vi "Begin.vi"(8 "error in":errorcluster) -> (0 "error out":errorcluster)   [LabVIEW 2019]
doc: "Called before other user functions, this VI can be used to open I/O refnums, load in file data, and do general program initialization. Notice that the <B>error out</B> terminal is simply used for data flow. Wiring it to other structures or subVIs ensures that this VI runs first."
uses:
  <vilib>/Rock Robotics/WPI/DriverStation/WPI_DriverStationRobotMode2.ctl
  <vilib>/Rock Robotics/WPI/Joystick/WPI_JoystickDeviceEnum.ctl
  <vilib>/Rock Robotics/SystemInterfaces/DIO/FPGA_DIOPWMChannel.ctl
  <vilib>/Rock Robotics/WPI/SafetyOutput/WPI_SafetyOutputConfigMenu.ctl
  <vilib>/Rock Robotics/WPI/Solenoid/WPI_SolenoidChannel.ctl
  <vilib>/Rock Robotics/SystemInterfaces/i2clib/i2c_bus.ctl
  <vilib>/Rock Robotics/WPI/Solenoid/WPI_SolenoidValue.ctl
  Robot Global Data.vi
  <vilib>/Rock Robotics/WPI/RobotDrive/WPI_RobotDriveOpen2MotorWithExistingMotors.vi
  <vilib>/Rock Robotics/WPI/MotorControl/WPI_MotorControlOpen SPARK.vi
  <vilib>/Rock Robotics/WPI/Solenoid/WPI_SolenoidOpenDouble.vi
  <vilib>/Rock Robotics/WPI/Solenoid/WPI_SolenoidSetEnum.vi
  <vilib>/Rock Robotics/Network Tables/NT Write Number.vi
  <vilib>/Rock Robotics/Network Tables/NT Write Boolean Array.vi
  <vilib>/Rock Robotics/Network Tables/NT Write Numeric Array.vi
panel:
  in  "Calibration Time (sec)":u32=4
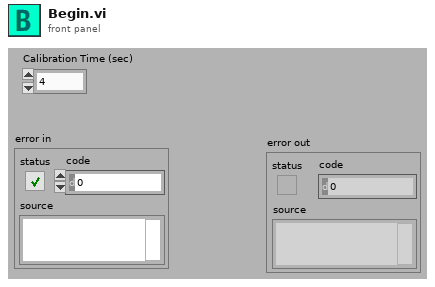
[diagram p1: front panel]
types:
  T1 = typedef "WPI_SolenoidChannel.ctl" = enum8{"Solenoid 0", "Solenoid 1", "Solenoid 2", "Solenoid 3", "Solenoid 4", "Solenoid 5", "Solenoid 6", "Solenoid 7", "Invalid"}
  T2 = typedef "WPI_SolenoidValue.ctl" = enum16{"Off", "On", "Forward", "Reverse"}
  T3 = typedef "WPI_SafetyOutputConfigMenu.ctl" = enum16{"Enable", "Disable"}
  T4 = typedef "i2c_bus.ctl" = enum16{"I2C On-Board", "I2C MXP", "Invalid"}
  T5 = typedef "FPGA_DIOPWMChannel.ctl" = enum8{"PWM 0", "PWM 1", "PWM 2", "PWM 3", "PWM 4", "PWM 5", "PWM 6", "PWM 7", "PWM 8", "PWM 9", "PWM MXP 0", "PWM MXP 1", "PWM MXP 2", "PWM MXP 3", "PWM MXP 4", "PWM MXP 5", "PWM MXP 6", "PWM MXP 7", "PWM MXP 8", "PWM MXP 9", "Invalid"}
  T6 = typedef "WPI_JoystickDeviceEnum.ctl" = enum16{"USB 0", "USB 1", "USB 2", "USB 3", "USB 4", "USB 5"}
  T7 = typedef "WPI_DriverStationRobotMode2.ctl" = enum16{"Autonomous Disabled", "Autonomous Enabled", "Teleop Disabled", "Teleop Enabled", "Disconnected", "Finish", "Test Disabled", "Test Enabled", "Emergency Stopped"}
  T8 = typedef "WPI_JoystickDevRef.ctl" = cluster{"Device":T6}
  T9 = typedef "WPI_MotorControlDeviceRef.ctl" = cluster{"DeviceStatus":errorcluster, "Type":T10, "PWM":cluster{"PWM Channel":T5, "DeadBand":T11}, "CAN":cluster{"Device Number":u8, "SetOutput VI Ref":variant, "GetOutput VI Ref":variant, "Enable VI Ref":variant, "Disable VI Ref":variant, "Data":variant}, "Invert":bool, "DIO PWM":cluster{"PWM \"Enable\" Channel":T5, "DIOChannel":T12, "PWM Rate":dbl}}
  T10 = typedef "WPI_MotorControlType.ctl" = enum16{"PWM", "CAN", "DIO PWM"}
  T11 = typedef "WPI_PWMDeadband.ctl" = cluster{"Name":string, "maxPositivePwm":i32, "minPositivePwm":i32, "centerPwm":i32, "maxNegativePwm":i32, "minNegativePwm":i32, "angularRange":u16}
  T12 = typedef "FPGA_DIOChannel.ctl" = enum8{"DIO 0", "DIO 1", "DIO 2", "DIO 3", "DIO 4", "DIO 5", "DIO 6", "DIO 7", "DIO 8", "DIO 9", "DIO MXP 0", "DIO MXP 1", "DIO MXP 2", "DIO MXP 3", "DIO MXP 4", "DIO MXP 5", "DIO MXP 6", "DIO MXP 7", "DIO MXP 8", "DIO MXP 9", "DIO MXP 10", "DIO MXP 11", "DIO MXP 12", "DIO MXP 13", "DIO MXP 14", "DIO MXP 15", "SPI Port CS1", "SPI Port CS2", "SPI Port CS3", "SPI Port MISO", "SPI Port MOSI", "Invalid"}
  T13 = typedef "WPI_RobotDriveDevRef.ctl" = cluster{"DevStatus":errorcluster, "Motors[]":T9[], "Square Inputs":bool, "Max Output":dbl}
  T14 = typedef "ADIS 16448 HW Configuration.ctl" = cluster{"SPI Clock Rate (Hz)":dbl, "IMU SPI Mode (3)":T15, "IMU Reset Pin":T12, "IMU SPI Bus":T16, "IMU Data Ready Pin":T12, "Stall Config":cluster{"Pow2BytesPerRead":u8, "StallTicks":u16, "CsToSclkTicks":u8}, "IMU Status LED Pin":T12}
  T15 = typedef "WPI_SPIMode.ctl" = enum16{"Mode 0 (Clk Idle Low,Sample on Leading)", "Mode 1 (Clk Idle Low,Sample on Trailing)", "Mode 2 (Clk Idle High,Sample on Leading)", "Mode 3 (Clk Idle High,Sample on Trailing)"}
  T16 = typedef "spi_bus.ctl" = enum16{"SPI On-Board, CS0", "SPI On-Board, CS1", "SPI On-Board, CS2", "SPI On-Board, CS3", "SPI MXP", "Invalid"}
  T17 = typedef "ADIS16448 Device Reference.ctl" = cluster{"DevStatus":errorcluster, "Hardware Config":T18, "Calibration Complete":refnum<notifier>, "Status FIFO":refnum<k33>, "Last Value Reference":refnum<data-value>, "Sychronous Process VI":T19, "Cmd FIFO":refnum<k33>, "Source":T20, "Data FIFO":refnum<k33>, "IMU Status LED Pin":T12, "Calibration Time":u32}
  T18 = typedef "ADIS16448 Hardware Configuration.ctl" = cluster{"SPI Clock Rate (Hz)":dbl, "IMU SPI Mode (3)":T15, "IMU Reset Pin":T12, "IMU SPI Bus":T16, "IMU Data Ready Pin":T12, "Stall Config":cluster{"Pow2BytesPerRead":u8, "StallTicks":u16, "CsToSclkTicks":u8}, "IMU Status LED Pin":T12}
  T19 = typedef "ADIS16448 Process.ctl" = refnum<vi>
  T20 = typedef "FPGA_CounterEncoderSourceConvertionLVSourceType.ctl" = cluster{"DevStatus":errorcluster, "AnalogTriggerMode?":bool, "DigitalMode":cluster{"DIO Channel":T21}, "AnalogTriggerMode":cluster{"AnalogTriggerIndex":T22, "OutputType":T23}}
  T21 = typedef "FPGA_DIODigitalSourceChannel.ctl" = enum8{"DIO 0", "DIO 1", "DIO 2", "DIO 3", "DIO 4", "DIO 5", "DIO 6", "DIO 7", "DIO 8", "DIO 9", "DIO MXP 0", "DIO MXP 1", "DIO MXP 2", "DIO MXP 3", "DIO MXP 4", "DIO MXP 5", "DIO MXP 6", "DIO MXP 7", "DIO MXP 8", "DIO MXP 9", "DIO MXP 10", "DIO MXP 11", "DIO MXP 12", "DIO MXP 13", "DIO MXP 14", "DIO MXP 15", "SPI Port CS1", "SPI Port CS2", "SPI Port CS3", "SPI Port MISO", "SPI Port MOSI", "Disabled"}
  T22 = typedef "FPGA_AnalogTriggerIndex.ctl" = enum8{"Trig 0", "Trig 1", "Trig 2", "Trig 3", "Trig 4", "Trig 5", "Trig 6", "Trig 7", "Invalid"}
  T23 = typedef "FPGA_AnalogTriggerOutType.ctl" = enum16{"InWindow", "TriggerState", "Rising", "Falling"}
  T24 = typedef "Color Sensor V3 DevRef.ctl" = cluster{"I2CDevRef":T25}
  T25 = typedef "WPI_I2CDevRef.ctl" = cluster{"DevStatus":errorcluster, "Device Address":u8, "Handle":i32, "I2C Bus":T4}
  T26 = typedef "WPI_SolenoidDevRef.ctl" = cluster{"DevStatus":errorcluster, "Pneumatics Control Module":u8, "Forward Solenoid Channel":T1, "Reverse Solenoid Channel":T1}
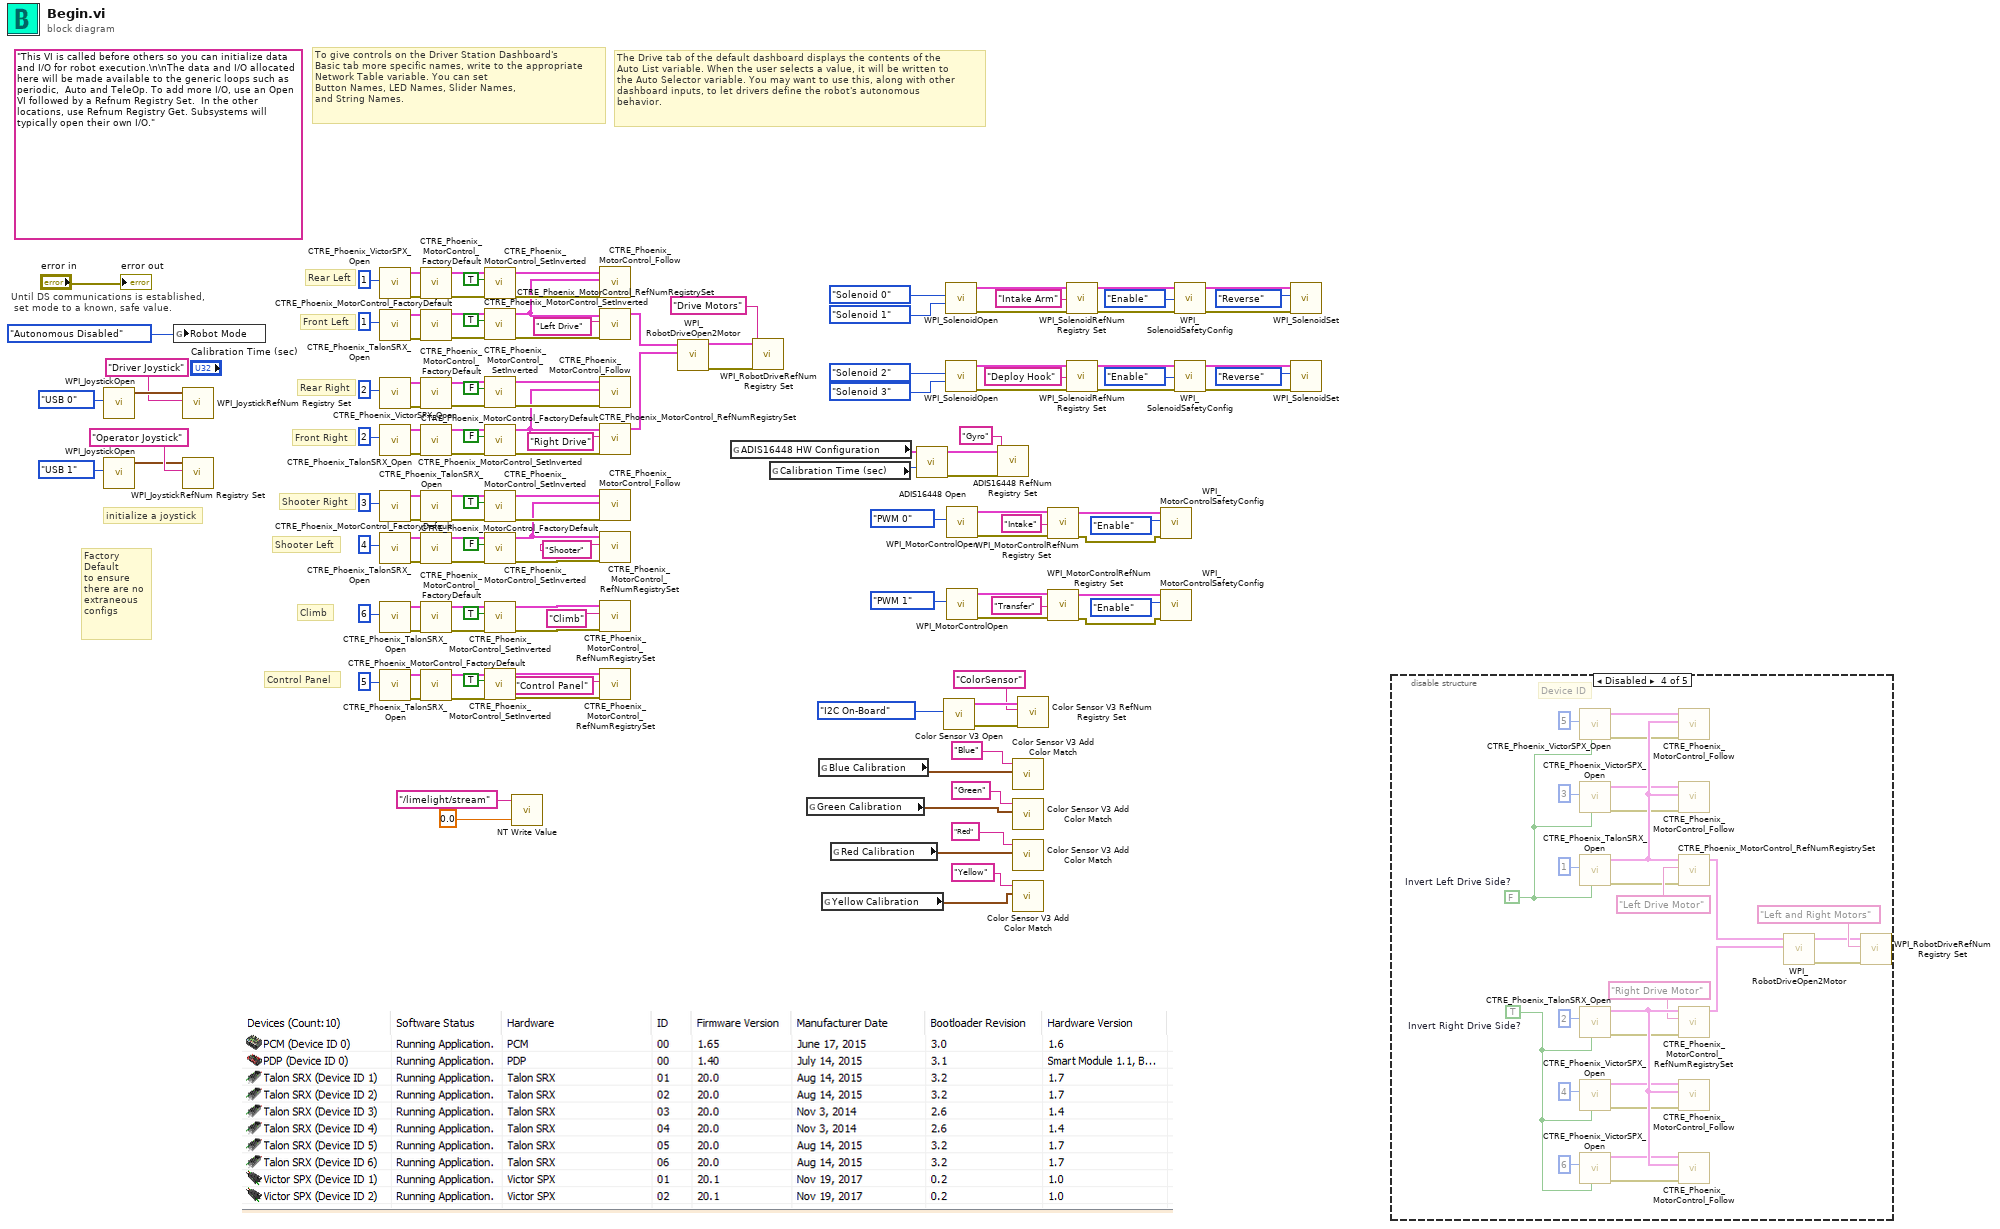
[diagram p0: block diagram]
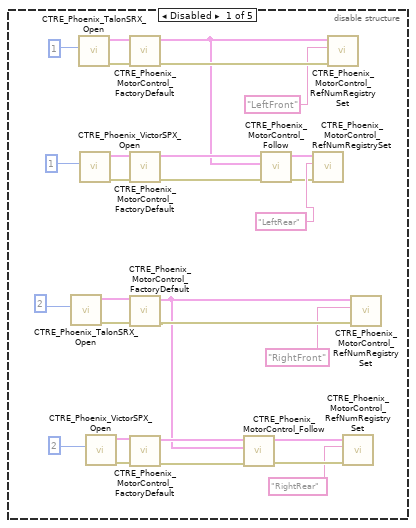
[diagram p2: hidden frame]
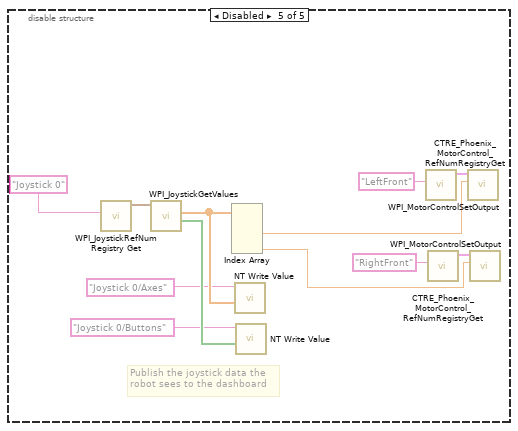
[diagram p5: hidden frame]
diagram:
  (unwired) "This VI is called before others so you can initialize data and I/O for robot execution.\n\nThe data and I/O allocated here will be made available to the generic loops such as periodic,  Auto and TeleOp. To add more I/O, use an Open VI followed by a Refnum Registry Set.  In the other locations, use Refnum Registry Get. Subsystems will typically open their own I/O."
  # "Climb"
  # "Control Panel"
  # "The Drive tab of the default dashboard displays the contents of the\nAuto List variable. When the user selects a value, it will be written to\nthe Auto Selector variable. You may want to use this, along with other\ndashboard inputs, to let drivers define the robot's autonomous\nbehavior."
  # "To give controls on the Driver Station Dashboard's\nBasic tab more specific names, write to the appropriate\nNetwork Table variable. You can set\nButton Names, LED Names, Slider Names,\nand String Names."
  # "Shooter Left"
  # "Shooter Right"
  # "Factory \nDefault \nto ensure \nthere are no \nextraneous \nconfigs"
  # "Front Right"
  # "Front Left"
  # "Rear Right"
  # "Rear Left"
  # "initialize a joystick"
  # "Until DS communications is established,\n set mode to a known, safe value."
  n1 = call <vilib>:"WPI_JoystickOpen.vi"("JoystickDevice"=WPI_JoystickDeviceEnum."USB 0") -> ("JoystickDevRef"=w120:T8)  [unwired: 10 in]
  n2 = call <vilib>:"WPI_JoystickOpen.vi"("JoystickDevice"=WPI_JoystickDeviceEnum."USB 1") -> ("JoystickDevRef"=w135:T8)  [unwired: 10 in]
  n3 = global write "Robot Global Data.vi" "Robot Mode"(WPI_DriverStationRobotMode2."Autonomous Disabled" ("Robot Mode")) -> ()
  n4 = call <vilib>:"WPI_JoystickRefNum Registry Set.vi"("refnum name"="Driver Joystick", "JoystickDevRef"=w120) -> ()  [unwired: 8 in, 2 out]
  n5 = call <vilib>:"WPI_JoystickRefNum Registry Set.vi"("refnum name"="Operator Joystick", "JoystickDevRef"=w135) -> ()  [unwired: 8 in, 2 out]
  n6 = call <vilib>:"CTRE_Phoenix_VictorSPX_Open.vi"("Device Number"=u8 1) -> ("error out"=w118:errorcluster, "CAN Talon SRX Ref"=w117:T9)  [unwired: 9 in]
  n7 = call <vilib>:"CTRE_Phoenix_TalonSRX_Open.vi"("Device Number"=u8 1) -> ("error out"=w115:errorcluster, "CAN Talon SRX Ref"=w116:T9)  [unwired: 9 in]
  n8 = call <vilib>:"CTRE_Phoenix_VictorSPX_Open.vi"("Device Number"=u8 2) -> ("error out"=w114:errorcluster, "CAN Talon SRX Ref"=w113:T9)  [unwired: 9 in]
  n9 = call <vilib>:"CTRE_Phoenix_TalonSRX_Open.vi"("Device Number"=u8 2) -> ("error out"=w112:errorcluster, "CAN Talon SRX Ref"=w111:T9)  [unwired: 9 in]
  n10 = call <vilib>:"CTRE_Phoenix_TalonSRX_Open.vi"("Device Number"=u8 3) -> ("error out"=w73:errorcluster, "CAN Talon SRX Ref"=w72:T9)  [unwired: 9 in]
  n11 = call <vilib>:"CTRE_Phoenix_TalonSRX_Open.vi"("Device Number"=u8 4) -> ("error out"=w71:errorcluster, "CAN Talon SRX Ref"=w70:T9)  [unwired: 9 in]
  n12 = call <vilib>:"CTRE_Phoenix_TalonSRX_Open.vi"("Device Number"=u8 6) -> ("error out"=w11:errorcluster, "CAN Talon SRX Ref"=w10:T9)  [unwired: 9 in]
  n13 = call <vilib>:"CTRE_Phoenix_TalonSRX_Open.vi"("Device Number"=u8 5) -> ("error out"=w41:errorcluster, "CAN Talon SRX Ref"=w40:T9)  [unwired: 9 in]
  n14 = call <vilib>:"CTRE_Phoenix_MotorControl_FactoryDefault.vi"("error in"=w118, "PhoenixMotorControlDevRef"=w117) -> ("error out"=w109:errorcluster, "PhoenixMotorControlDevRef"=w108:T9)  [unwired: 8 in]
  n15 = call <vilib>:"CTRE_Phoenix_MotorControl_FactoryDefault.vi"("error in"=w115, "PhoenixMotorControlDevRef"=w116) -> ("error out"=w103:errorcluster, "PhoenixMotorControlDevRef"=w104:T9)  [unwired: 8 in]
  n16 = call <vilib>:"CTRE_Phoenix_MotorControl_FactoryDefault.vi"("error in"=w114, "PhoenixMotorControlDevRef"=w113) -> ("error out"=w99:errorcluster, "PhoenixMotorControlDevRef"=w98:T9)  [unwired: 8 in]
  n17 = call <vilib>:"CTRE_Phoenix_MotorControl_FactoryDefault.vi"("error in"=w112, "PhoenixMotorControlDevRef"=w111) -> ("error out"=w94:errorcluster, "PhoenixMotorControlDevRef"=w93:T9)  [unwired: 8 in]
  n18 = call <vilib>:"CTRE_Phoenix_MotorControl_FactoryDefault.vi"("error in"=w73, "PhoenixMotorControlDevRef"=w72) -> ("error out"=w67:errorcluster, "PhoenixMotorControlDevRef"=w68:T9)  [unwired: 8 in]
  n19 = call <vilib>:"CTRE_Phoenix_MotorControl_FactoryDefault.vi"("error in"=w71, "PhoenixMotorControlDevRef"=w70) -> ("error out"=w62:errorcluster, "PhoenixMotorControlDevRef"=w63:T9)  [unwired: 8 in]
  n20 = call <vilib>:"CTRE_Phoenix_MotorControl_FactoryDefault.vi"("error in"=w11, "PhoenixMotorControlDevRef"=w10) -> ("error out"=w7:errorcluster, "PhoenixMotorControlDevRef"=w8:T9)  [unwired: 8 in]
  n21 = call <vilib>:"CTRE_Phoenix_MotorControl_FactoryDefault.vi"("error in"=w41, "PhoenixMotorControlDevRef"=w40) -> ("error out"=w37:errorcluster, "PhoenixMotorControlDevRef"=w38:T9)  [unwired: 8 in]
  n22 = call <vilib>:"CTRE_Phoenix_MotorControl_SetInverted.vi"("error in (no error)"=w109, "Invert?"=TRUE, "PhoenixMotorControlDevRef"=w108) -> ("error out"=w106:errorcluster, "PhoenixMotorControlDevRef"=w107:T9)  [unwired: 7 in]
  n23 = call <vilib>:"CTRE_Phoenix_MotorControl_SetInverted.vi"("error in (no error)"=w103, "Invert?"=TRUE, "PhoenixMotorControlDevRef"=w104) -> ("error out"=w102:errorcluster, "PhoenixMotorControlDevRef"=w101:T9)  [unwired: 7 in]
  n24 = call <vilib>:"CTRE_Phoenix_MotorControl_SetInverted.vi"("error in (no error)"=w99, "Invert?"=FALSE, "PhoenixMotorControlDevRef"=w98) -> ("error out"=w96:errorcluster, "PhoenixMotorControlDevRef"=w97:T9)  [unwired: 7 in]
  n25 = call <vilib>:"CTRE_Phoenix_MotorControl_SetInverted.vi"("error in (no error)"=w94, "Invert?"=FALSE, "PhoenixMotorControlDevRef"=w93) -> ("error out"=w91:errorcluster, "PhoenixMotorControlDevRef"=w92:T9)  [unwired: 7 in]
  n26 = call <vilib>:"CTRE_Phoenix_MotorControl_SetInverted.vi"("error in (no error)"=w67, "Invert?"=TRUE, "PhoenixMotorControlDevRef"=w68) -> ("error out"=w66:errorcluster, "PhoenixMotorControlDevRef"=w65:T9)  [unwired: 7 in]
  n27 = call <vilib>:"CTRE_Phoenix_MotorControl_SetInverted.vi"("error in (no error)"=w62, "Invert?"=FALSE, "PhoenixMotorControlDevRef"=w63) -> ("error out"=w61:errorcluster, "PhoenixMotorControlDevRef"=w60:T9)  [unwired: 7 in]
  n28 = call <vilib>:"CTRE_Phoenix_MotorControl_SetInverted.vi"("error in (no error)"=w7, "Invert?"=TRUE, "PhoenixMotorControlDevRef"=w8) -> ("error out"=w6:errorcluster, "PhoenixMotorControlDevRef"=w5:T9)  [unwired: 7 in]
  n29 = call <vilib>:"CTRE_Phoenix_MotorControl_SetInverted.vi"("error in (no error)"=w37, "Invert?"=TRUE, "PhoenixMotorControlDevRef"=w38) -> ("error out"=w36:errorcluster, "PhoenixMotorControlDevRef"=w35:T9)  [unwired: 7 in]
  n30 = call-poly <vilib>:"NT Write Value.vi"("Numeric"=0.0, "Name"="/limelight/stream") -> ()  [unwired: 9 in, 1 out]
  n31 = call <vilib>:"CTRE_Phoenix_MotorControl_Follow.vi"("error in (no error)"=w106, "Master Controller to Follow"=w101, "PhoenixMotorControlDevRef"=w107) -> ()  [unwired: 7 in, 2 out]
  n32 = call <vilib>:"CTRE_Phoenix_MotorControl_RefNumRegistrySet.vi"("error in (no error)"=w102, "refnum name"="Left Drive", "PhoenixMotorControlDevRef"=w101) -> ("PhoenixMotorControlDevRef"=w128:T9)  [unwired: 7 in, 1 out]
  n33 = call <vilib>:"CTRE_Phoenix_MotorControl_Follow.vi"("error in (no error)"=w96, "Master Controller to Follow"=w92, "PhoenixMotorControlDevRef"=w97) -> ()  [unwired: 7 in, 2 out]
  n34 = call <vilib>:"CTRE_Phoenix_MotorControl_RefNumRegistrySet.vi"("error in (no error)"=w91, "refnum name"="Right Drive", "PhoenixMotorControlDevRef"=w92) -> ("PhoenixMotorControlDevRef"=w127:T9)  [unwired: 7 in, 1 out]
  n35 = call <vilib>:"CTRE_Phoenix_MotorControl_Follow.vi"("error in (no error)"=w66, "Master Controller to Follow"=w60, "PhoenixMotorControlDevRef"=w65) -> ()  [unwired: 7 in, 2 out]
  n36 = call <vilib>:"CTRE_Phoenix_MotorControl_RefNumRegistrySet.vi"("error in (no error)"=w61, "refnum name"="Shooter", "PhoenixMotorControlDevRef"=w60) -> ()  [unwired: 7 in, 2 out]
  n37 = call <vilib>:"CTRE_Phoenix_MotorControl_RefNumRegistrySet.vi"("error in (no error)"=w6, "refnum name"="Climb", "PhoenixMotorControlDevRef"=w5) -> ()  [unwired: 7 in, 2 out]
  n38 = call <vilib>:"CTRE_Phoenix_MotorControl_RefNumRegistrySet.vi"("error in (no error)"=w36, "refnum name"="Control Panel", "PhoenixMotorControlDevRef"=w35) -> ()  [unwired: 7 in, 2 out]
  n39 = call-poly <vilib>:"WPI_RobotDriveOpen2Motor.vi"("Right Motor Dev Ref"=w127, "Left Motor Dev Ref"=w128) -> ("error out"=w123:errorcluster, "RobotDriveDevRef"=w124:T13)  [unwired: 8 in]
  n40 = global read "Robot Global Data.vi" "ADIS16448 HW Configuration"() -> (w59:T14)
  n41 = call <vilib>:"WPI_RobotDriveRefNum Registry Set.vi"("error in (no error)"=w123, "refnum name"="Drive Motors", "RobotDriveDevRef"=w124) -> ()  [unwired: 7 in, 2 out]
  n42 = global read "Robot Global Data.vi" "Calibration Time (sec)"() -> (w58:u32)
  n43 = global read "Robot Global Data.vi" "Green Calibration"() -> (w3:cluster{"R":dbl, "G":dbl, "B":dbl})
  n44 = global read "Robot Global Data.vi" "Blue Calibration"() -> (w4:cluster{"R":dbl, "G":dbl, "B":dbl})
  n45 = global read "Robot Global Data.vi" "Yellow Calibration"() -> (w1:cluster{"R":dbl, "G":dbl, "B":dbl})
  n46 = global read "Robot Global Data.vi" "Red Calibration"() -> (w2:cluster{"R":dbl, "G":dbl, "B":dbl})
  n47 = call <vilib>:"ADIS16448 Open.vi"("Initial Calibration Time (sec)"=w58, "Hardware Config"=w59) -> ("error out"=w56:errorcluster, "ADIS16448DevRef"=w57:T17)  [unwired: 8 in]
  n48 = call <vilib>:"Color Sensor V3 Open.vi"("I2C Bus"=i2c_bus."I2C On-Board") -> ("error out"=w32:errorcluster, "ColorSensorDevRef"=w33:T24)  [unwired: 9 in]
  n49 = call-poly <vilib>:"WPI_SolenoidOpen.vi"("Reverse Solenoid Channel"=WPI_SolenoidChannel."Solenoid 1" ("Solenoid Channel"), "Forward Solenoid Channel"=WPI_SolenoidChannel."Solenoid 0" ("Solenoid Channel")) -> ("error out"=w51:errorcluster, "SolenoidDevRef"=w54:T26)  [unwired: 8 in]
  n50 = call-poly <vilib>:"WPI_SolenoidOpen.vi"("Reverse Solenoid Channel"=WPI_SolenoidChannel."Solenoid 3" ("Solenoid Channel"), "Forward Solenoid Channel"=WPI_SolenoidChannel."Solenoid 2" ("Solenoid Channel")) -> ("error out"=w18:errorcluster, "SolenoidDevRef"=w15:T26)  [unwired: 8 in]
  n51 = call-poly <vilib>:"WPI_MotorControlOpen.vi"("PWM Channel"=FPGA_DIOPWMChannel."PWM 0") -> ("error out"=w85:errorcluster, "MotorControlDeviceRef"=w89:T9)  [unwired: 9 in]
  n52 = call-poly <vilib>:"WPI_MotorControlOpen.vi"("PWM Channel"=FPGA_DIOPWMChannel."PWM 1") -> ("error out"=w82:errorcluster, "MotorControlDeviceRef"=w78:T9)  [unwired: 9 in]
  n53 = call <vilib>:"ADIS16448 RefNum Registry Set.vi"("error in (no error)"=w56, "refnum name"="Gyro", "ADIS16448DevRef"=w57) -> ()  [unwired: 7 in, 2 out]
  n54 = call <vilib>:"Color Sensor V3 Add Color Match.vi"("Color"=w4, "Name"="Blue") -> ()  [unwired: 10 in]
  n55 = call <vilib>:"Color Sensor V3 Add Color Match.vi"("Color"=w3, "Name"="Green") -> ()  [unwired: 10 in]
  n56 = call <vilib>:"Color Sensor V3 Add Color Match.vi"("Color"=w2, "Name"="Red") -> ()  [unwired: 10 in]
  n57 = call <vilib>:"Color Sensor V3 Add Color Match.vi"("Color"=w1, "Name"="Yellow") -> ()  [unwired: 10 in]
  n58 = call <vilib>:"Color Sensor V3 RefNum Registry Set.vi"("error in (no error)"=w32, "refnum name"="ColorSensor", "ColorSensorDevRef"=w33) -> ()  [unwired: 7 in, 2 out]
  n59 = call <vilib>:"WPI_MotorControlRefNum Registry Set.vi"("error in (no error)"=w85, "refnum name"="Intake", "MotorControlDevRef"=w89) -> ("error out"=w84:errorcluster, "MotorControlDevRef"=w88:T9)  [unwired: 7 in]
  n60 = call <vilib>:"WPI_MotorControlRefNum Registry Set.vi"("error in (no error)"=w82, "refnum name"="Transfer", "MotorControlDevRef"=w78) -> ("error out"=w83:errorcluster, "MotorControlDevRef"=w79:T9)  [unwired: 7 in]
  n61 = call <vilib>:"WPI_SolenoidRefNum Registry Set.vi"("error in (no error)"=w51, "refnum name"="Intake Arm", "SolenoidDevRef"=w54) -> ("error out"=w50:errorcluster, "SolenoidDevRef"=w53:T26)  [unwired: 7 in]
  n62 = call <vilib>:"WPI_SolenoidRefNum Registry Set.vi"("error in (no error)"=w18, "refnum name"="Deploy Hook", "SolenoidDevRef"=w15) -> ("error out"=w19:errorcluster, "SolenoidDevRef"=w16:T26)  [unwired: 7 in]
  n63 = call <vilib>:"WPI_MotorControlSafetyConfig.vi"("error in (no error)"=w84, "mode"=WPI_SafetyOutputConfigMenu."Enable", "MotorControlDevRef"=w88) -> ()  [unwired: 7 in, 2 out]
  n64 = call <vilib>:"WPI_MotorControlSafetyConfig.vi"("error in (no error)"=w83, "mode"=WPI_SafetyOutputConfigMenu."Enable", "MotorControlDevRef"=w79) -> ()  [unwired: 7 in, 2 out]
  n65 = call <vilib>:"WPI_SolenoidSafetyConfig.vi"("error in (no error)"=w50, "mode"=WPI_SafetyOutputConfigMenu."Enable", "SolenoidDevRef"=w53) -> ("error out"=w49:errorcluster, "SolenoidDevRef"=w52:T26)  [unwired: 7 in]
  n66 = call <vilib>:"WPI_SolenoidSafetyConfig.vi"("error in (no error)"=w19, "mode"=WPI_SafetyOutputConfigMenu."Enable", "SolenoidDevRef"=w16) -> ("error out"=w20:errorcluster, "SolenoidDevRef"=w17:T26)  [unwired: 7 in]
  n67 = call-poly <vilib>:"WPI_SolenoidSet.vi"("error in (no error)"=w49, "Value"=WPI_SolenoidValue."Reverse", "SolenoidDevRef"=w52) -> ()  [unwired: 7 in, 2 out]
  n68 = call-poly <vilib>:"WPI_SolenoidSet.vi"("error in (no error)"=w20, "Value"=WPI_SolenoidValue."Reverse", "SolenoidDevRef"=w17) -> ()  [unwired: 7 in, 2 out]
  n69 = disable-structure shown="Disabled" {
    frame Disabled {
      n70 = call <vilib>:"CTRE_Phoenix_TalonSRX_Open.vi"("Device Number"=u8 2) -> ("error out"=w162:errorcluster, "CAN Talon SRX Ref"=w152:T9)  [unwired: 9 in]
      n71 = call <vilib>:"CTRE_Phoenix_TalonSRX_Open.vi"("Device Number"=u8 1) -> ("error out"=w160:errorcluster, "CAN Talon SRX Ref"=w150:T9)  [unwired: 9 in]
      n72 = call <vilib>:"CTRE_Phoenix_VictorSPX_Open.vi"("Device Number"=u8 1) -> ("error out"=w158:errorcluster, "CAN Talon SRX Ref"=w156:T9)  [unwired: 9 in]
      n73 = call <vilib>:"CTRE_Phoenix_VictorSPX_Open.vi"("Device Number"=u8 2) -> ("error out"=w164:errorcluster, "CAN Talon SRX Ref"=w154:T9)  [unwired: 9 in]
      n74 = call <vilib>:"CTRE_Phoenix_MotorControl_FactoryDefault.vi"("error in"=w160, "PhoenixMotorControlDevRef"=w150) -> ("error out"=w161:errorcluster, "PhoenixMotorControlDevRef"=w151:T9)  [unwired: 8 in]
      n75 = call <vilib>:"CTRE_Phoenix_MotorControl_FactoryDefault.vi"("error in"=w158, "PhoenixMotorControlDevRef"=w156) -> ("error out"=w159:errorcluster, "PhoenixMotorControlDevRef"=w157:T9)  [unwired: 8 in]
      n76 = call <vilib>:"CTRE_Phoenix_MotorControl_FactoryDefault.vi"("error in"=w162, "PhoenixMotorControlDevRef"=w152) -> ("error out"=w163:errorcluster, "PhoenixMotorControlDevRef"=w153:T9)  [unwired: 8 in]
      n77 = call <vilib>:"CTRE_Phoenix_MotorControl_FactoryDefault.vi"("error in"=w164, "PhoenixMotorControlDevRef"=w154) -> ("error out"=w165:errorcluster, "PhoenixMotorControlDevRef"=w155:T9)  [unwired: 8 in]
      n78 = call <vilib>:"CTRE_Phoenix_MotorControl_Follow.vi"("error in (no error)"=w165, "Master Controller to Follow"=w153, "PhoenixMotorControlDevRef"=w155) -> ("error out"=w148:errorcluster, "PhoenixMotorControlDevRef"=w149:T9)  [unwired: 7 in]
      n79 = call <vilib>:"CTRE_Phoenix_MotorControl_Follow.vi"("error in (no error)"=w159, "Master Controller to Follow"=w151, "PhoenixMotorControlDevRef"=w157) -> ("error out"=w140:errorcluster, "PhoenixMotorControlDevRef"=w141:T9)  [unwired: 7 in]
      n80 = call <vilib>:"CTRE_Phoenix_MotorControl_RefNumRegistrySet.vi"("error in (no error)"=w140, "refnum name"="LeftRear", "PhoenixMotorControlDevRef"=w141) -> ()  [unwired: 7 in, 2 out]
      n81 = call <vilib>:"CTRE_Phoenix_MotorControl_RefNumRegistrySet.vi"("error in (no error)"=w161, "refnum name"="LeftFront", "PhoenixMotorControlDevRef"=w151) -> ()  [unwired: 7 in, 2 out]
      n82 = call <vilib>:"CTRE_Phoenix_MotorControl_RefNumRegistrySet.vi"("error in (no error)"=w148, "refnum name"="RightRear", "PhoenixMotorControlDevRef"=w149) -> ()  [unwired: 7 in, 2 out]
      n83 = call <vilib>:"CTRE_Phoenix_MotorControl_RefNumRegistrySet.vi"("error in (no error)"=w163, "refnum name"="RightFront", "PhoenixMotorControlDevRef"=w153) -> ()  [unwired: 7 in, 2 out]
    }
    frame Enabled {
    }
    frame Disabled {
    }
    frame Disabled {
      w192 = FALSE  # Invert Left Drive Side?
      w191 = TRUE  # Invert Right Drive Side?
      # "Device ID"
      n84 = call <vilib>:"CTRE_Phoenix_VictorSPX_Open.vi"("Invert"=w192, "Device Number"=u8 5) -> ("error out"=w182:errorcluster, "CAN Talon SRX Ref"=w183:T9)  [unwired: 8 in]
      n85 = call <vilib>:"CTRE_Phoenix_VictorSPX_Open.vi"("Invert"=w192, "Device Number"=u8 3) -> ("error out"=w181:errorcluster, "CAN Talon SRX Ref"=w184:T9)  [unwired: 8 in]
      n86 = call <vilib>:"CTRE_Phoenix_TalonSRX_Open.vi"("Invert"=w192, "Device Number"=u8 1) -> ("error out"=w172:errorcluster, "CAN Talon SRX Ref"=w185:T9)  [unwired: 8 in]
      n87 = call <vilib>:"CTRE_Phoenix_TalonSRX_Open.vi"("Invert"=w191, "Device Number"=u8 2) -> ("error out"=w173:errorcluster, "CAN Talon SRX Ref"=w180:T9)  [unwired: 8 in]
      n88 = call <vilib>:"CTRE_Phoenix_VictorSPX_Open.vi"("Invert"=w191, "Device Number"=u8 4) -> ("error out"=w176:errorcluster, "CAN Talon SRX Ref"=w177:T9)  [unwired: 8 in]
      n89 = call <vilib>:"CTRE_Phoenix_VictorSPX_Open.vi"("Invert"=w191, "Device Number"=u8 6) -> ("error out"=w179:errorcluster, "CAN Talon SRX Ref"=w178:T9)  [unwired: 8 in]
      n90 = call <vilib>:"CTRE_Phoenix_MotorControl_Follow.vi"("error in (no error)"=w182, "Master Controller to Follow"=w185, "PhoenixMotorControlDevRef"=w183) -> ()  [unwired: 7 in, 2 out]
      n91 = call <vilib>:"CTRE_Phoenix_MotorControl_Follow.vi"("error in (no error)"=w181, "Master Controller to Follow"=w185, "PhoenixMotorControlDevRef"=w184) -> ()  [unwired: 7 in, 2 out]
      n92 = call <vilib>:"CTRE_Phoenix_MotorControl_RefNumRegistrySet.vi"("error in (no error)"=w172, "refnum name"="Left Drive Motor", "PhoenixMotorControlDevRef"=w185) -> ("PhoenixMotorControlDevRef"=w186:T9)  [unwired: 7 in, 1 out]
      n93 = call <vilib>:"CTRE_Phoenix_MotorControl_RefNumRegistrySet.vi"("error in (no error)"=w173, "refnum name"="Right Drive Motor", "PhoenixMotorControlDevRef"=w180) -> ("PhoenixMotorControlDevRef"=w187:T9)  [unwired: 7 in, 1 out]
      n94 = call <vilib>:"CTRE_Phoenix_MotorControl_Follow.vi"("error in (no error)"=w176, "Master Controller to Follow"=w180, "PhoenixMotorControlDevRef"=w177) -> ()  [unwired: 7 in, 2 out]
      n95 = call <vilib>:"CTRE_Phoenix_MotorControl_Follow.vi"("error in (no error)"=w179, "Master Controller to Follow"=w180, "PhoenixMotorControlDevRef"=w178) -> ()  [unwired: 7 in, 2 out]
      n96 = call-poly <vilib>:"WPI_RobotDriveOpen2Motor.vi"("Right Motor Dev Ref"=w187, "Left Motor Dev Ref"=w186) -> ("error out"=w188:errorcluster, "RobotDriveDevRef"=w189:T13)  [unwired: 8 in]
      n97 = call <vilib>:"WPI_RobotDriveRefNum Registry Set.vi"("error in (no error)"=w188, "refnum name"="Left and Right Motors", "RobotDriveDevRef"=w189) -> ()  [unwired: 7 in, 2 out]
    }
    frame Disabled {
      # "Publish the joystick data the\nrobot sees to the dashboard"
      n98 = call <vilib>:"WPI_JoystickRefNum Registry Get.vi"("refnum name"="Joystick 0") -> ("JoystickDevRef"=w194:T8)  [unwired: 1 in, 9 out]
      n99 = call <vilib>:"WPI_JoystickGetValues.vi"("JoystickDevRef"=w194) -> ("Buttons"=w198:bool[], "Axes"=w197:dbl[])  [unwired: 6 in, 3 out]
      n100 = Index Array(array=w197) -> (element #2=w201:dbl, element #4=w204:dbl)  [unwired: 4 in, 2 out]
      n101 = call-poly <vilib>:"NT Write Value.vi"("Numeric Array"=w197, "Name"="Joystick 0/Axes") -> ()  [unwired: 9 in, 1 out]
      n102 = call-poly <vilib>:"NT Write Value.vi"("Boolean Array"=w198, "Name"="Joystick 0/Buttons") -> ()  [unwired: 9 in, 1 out]
      n103 = call <vilib>:"CTRE_Phoenix_MotorControl_RefNumRegistryGet.vi"("refnum name"="LeftFront") -> ("PhoenixMotorControlDevRef"=w200:T9)  [unwired: 9 in, 1 out]
      n104 = call <vilib>:"CTRE_Phoenix_MotorControl_RefNumRegistryGet.vi"("refnum name"="RightFront") -> ("PhoenixMotorControlDevRef"=w203:T9)  [unwired: 9 in, 1 out]
      n105 = call <vilib>:"WPI_MotorControlSetOutput.vi"("Output"=w201, "MotorControlDevRef"=w200) -> ()  [unwired: 7 in, 3 out]
      n106 = call <vilib>:"WPI_MotorControlSetOutput.vi"("Output"=w204, "MotorControlDevRef"=w203) -> ()  [unwired: 7 in, 3 out]
    }
  }
  "error out" <- "error in"
